vi "smart_get.vi"(2 "Input Image":T4, 3 "Cluster":T3) -> (0 "Image Out":T4, 1 "Acquired Buffer Number":i32)   [LabVIEW 2015]
uses:
  <vilib>/vision/Image Controls.llb/IMAQ Image.ctl
  <vilib>/vision/Avi1.llb/AviRefnum.ctl
  <vilib>/userdefined/High Color/IMAQdx.ctl
  <vilib>/vision/driver/NI_Vision_Acquisition_Software.lvlib
  <vilib>/vision/NI_Vision_Development_Module.lvlib
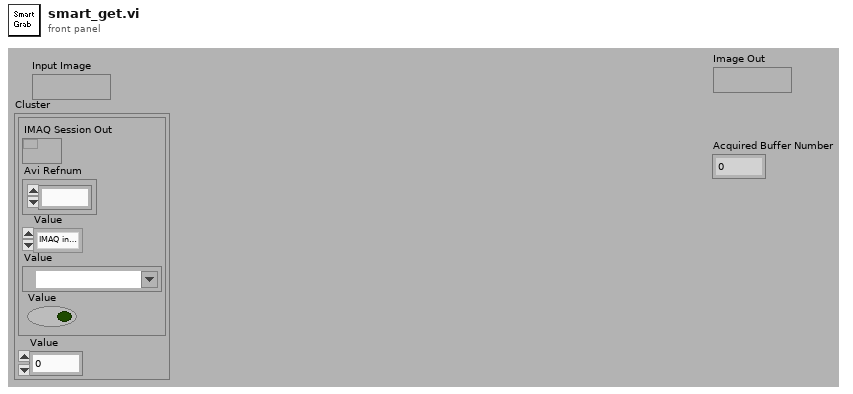
[diagram p1: front panel]
types:
  T1 = typedef "AviRefnum.ctl" = refnum<k1>
  T2 = typedef "IMAQdx.ctl" = refnum<k21>
  T3 = cluster{cluster{"IMAQ Session Out":refnum<k11>, "Avi Refnum":T1, "Value":enum32{"IMAQ interface", "IMAQdx interface", "AVI file"}, "Value":T2, "Value":bool}, "Value":i32}
  T4 = typedef "IMAQ Image.ctl" = refnum<image>
  T5 = typedef "Image Type" = u32
  T6 = cluster{"IMAQ Session Out":refnum<k11>, "Avi Refnum":T1, "Value":enum32{"IMAQ interface", "IMAQdx interface", "AVI file"}, "Value":T2, "Value":bool}
  T7 = enum32{"IMAQ interface", "IMAQdx interface", "AVI file"}
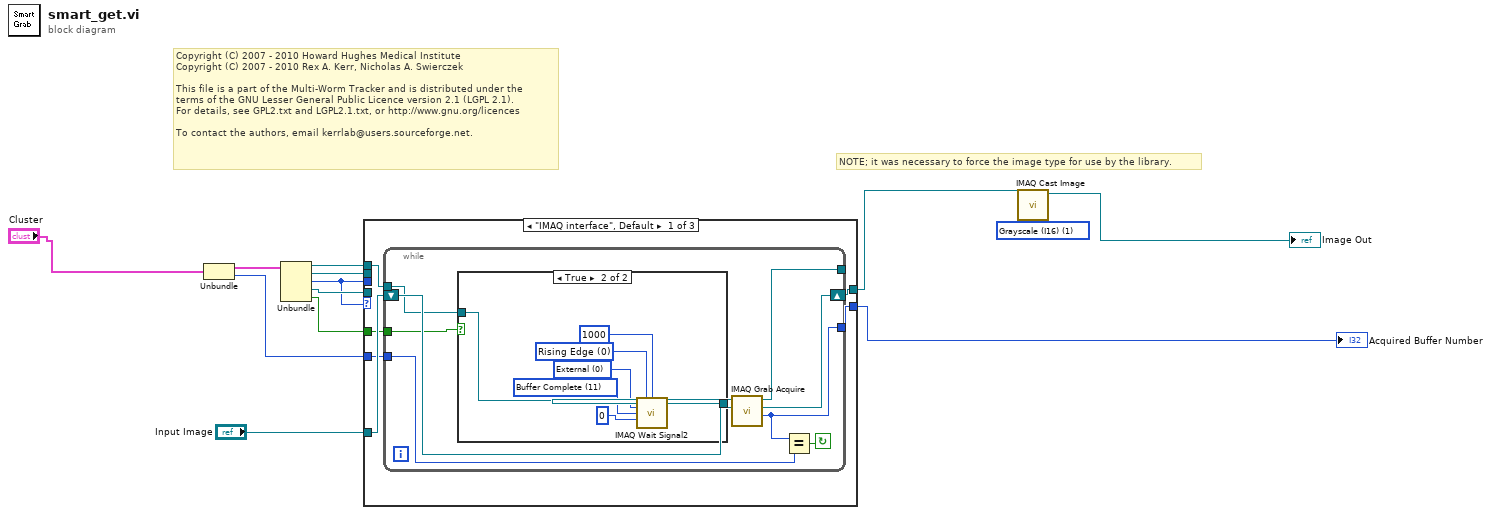
[diagram p0: block diagram]
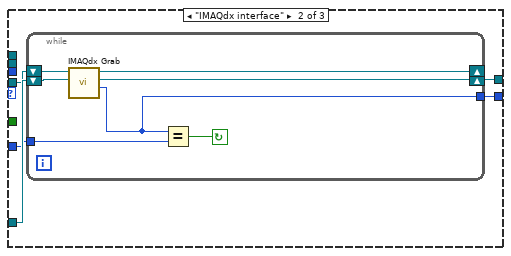
[diagram p3: hidden frame]
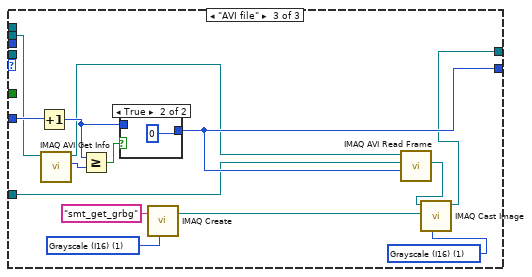
[diagram p4: hidden frame]
diagram:
  w4 = T5 1 items=["Grayscale (U8)", "Grayscale (I16)", "Grayscale (SGL)", "Complex (CSG)", "RGB (U32)", "HSL (U32)", "RGB (U64)"] ("Image Type")
  # "NOTE; it was necessary to force the image type for use by the library."
  # "Copyright (C) 2007 - 2010 Howard Hughes Medical Institute\nCopyright (C) 2007 - 2010 Rex A. Kerr, Nicholas A. Swierczek\n \nThis file is a part of the Multi-Worm Tracker and is distributed under the\nterms of the GNU Lesser General Public Licence version 2.1 (LGPL 2.1).\nFor details, see GPL2.txt and LGPL2.1.txt, or http://www.gnu.org/licences\n \nTo contact the authors, email kerrlab@users.sourceforge.net."
  n1 = Unbundle("Cluster") -> (w7:T6, "Value"=w11:i32)
  n2 = Unbundle(w7) -> ("IMAQ Session Out"=w13:refnum<k11>, "Avi Refnum"=w5:T1, "Value"=w3:T7, "Value"=w6:T2, "Value"=w1:bool)
  n3 = case shown="\"IMAQ interface\", Default" w3 {
    tunnel: w6 -> [_ w39 _]
    tunnel: w13 -> [w19 _ _]
    tunnel: "Input Image" -> [w18 w41 w56]
    tunnel: w11 -> [w17 w40 w62]
    tunnel: [w16 w38 w54] -> w8
    tunnel: [w15 w37 w58] -> w10
    tunnel: w3 -> [_ _ _]
    tunnel: w5 -> [_ _ w49]
    tunnel: w1 -> [w14 _ _]
    frame "IMAQ interface", Default {
      n4 = while {
        tunnel: [w26] -> _
        tunnel: [w25] -> w15
        tunnel: w19 -> [w22]
        tunnel: w17 -> [w23]
        shift-right: [w27] -> w16
        shift-left: w18 -> [w24]
        tunnel: w14 -> [w20]
        stop <- w28 continue-if-true
        n5 = case shown="True" w20 {
          tunnel: w22 -> [w29 w35]
          tunnel: [w29 w36] -> w21
          frame False {
          }
          frame True {
            w31 = u32 0 items=["Rising Edge", "Falling Edge"] ("Signal polarity")
            w32 = u32 0 items=["External", "RTSI ", "ISO In", "ISO Out", "Status"] ("Signal Type")
            w33 = u32 11 items=["Acquisition in progress"=15, "Acquisition done"=8, "Frame start"=9, "Frame done"=10, "Buffer Complete"=11] ("Status Signal")
            n6 = call <vilib>:"IMAQ Wait Signal2.vi"("IMAQ Session In"=w35, "Signal polarity"=w31, "Timeout (ms)"=u32 1000, "Signal Type"=w32, "Status Signal"=w33, "Signal Number"=u32 0) -> ("IMAQ Session Out"=w36:refnum<k11>)  [unwired: 8 in, 1 out]
          }
        }
        n7 = call <vilib>:"IMAQ Grab Acquire.vi"("Image In"=w24, "IMAQ Session In"=w21) -> ("Acquired Buffer Number"=w25:u32, "Image Out"=w27:T4, "IMAQ Session Out"=w26:refnum<k11>)  [unwired: 6 in, 1 out]
        n8 = Equal?(x=w25, y=w23) -> (x = y?=w28:bool)
      }
    }
    frame "IMAQdx interface" {
      n9 = while {
        tunnel: [w45] -> w37
        tunnel: w40 -> [w42]
        shift-right: [w47] -> w38
        shift-left: w41 -> [w43]
        shift-right: [w46] -> _
        shift-left: w39 -> [w44]
        stop <- w48 continue-if-true
        n10 = call <vilib>:"IMAQdx Grab.vi"("Image In"=w43, "Session In"=w44) -> ("Buffer Number Out"=w45:u32, "Image Out"=w47:T4, "Session Out"=w46:T2)  [unwired: 6 in, 1 out]
        n11 = Equal?(x=w45, y=w42) -> (x = y?=w48:bool)
      }
    }
    frame "AVI file" {
      w52 = T5 1 items=["Grayscale (U8)", "Grayscale (I16)", "Grayscale (SGL)", "Complex (CSG)", "RGB (U32)", "HSL (U32)", "RGB (U64)"] ("Image Type")
      w53 = T5 1 items=["Grayscale (U8)", "Grayscale (I16)", "Grayscale (SGL)", "Complex (CSG)", "RGB (U32)", "HSL (U32)", "RGB (U64)"] ("Image Type")
      n12 = Increment(x=w62) -> (x+1=w60:i32)
      n13 = call "IMAQ AVI Get Info"("Avi Refnum"=w49) -> ("Number of Frames"=w61:u32, "Avi Refnum (duplicate)"=w57:T1)  [unwired: 6 in, 3 out]
      n14 = Greater Or Equal?(x=w60, y=w61) -> (x >= y?=w59:bool)
      n15 = case shown="True" w59 {
        tunnel: w60 -> [w63 _]
        tunnel: [w63 0] -> w58
        frame False {
        }
        frame True {
        }
      }
      n16 = call "IMAQ Create"("Image Name"="smt_get_grbg", "Image Type"=w52) -> ("New Image"=w50:T4)  [unwired: 3 in, 1 out]
      n17 = call "IMAQ AVI Read Frame"("Frame Number"=w58, "Image"=w56, "Avi Refnum"=w57) -> ("Image Out"=w55:T4)  [unwired: 5 in, 3 out]
      n18 = call "IMAQ Cast Image"("Image Type"=w53, "Image Dst"=w50, "Image Src"=w55) -> ("Image Dst Out"=w54:T4)  [unwired: 7 in, 1 out]
    }
  }
  "Acquired Buffer Number" <- w10
  n19 = call "IMAQ Cast Image"("Image Type"=w4, "Image Src"=w8) -> ("Image Dst Out"=→"Image Out":T4)  [unwired: 8 in, 1 out]
